vi "Monitor DI Port 1.vi"(8 "Error in":errorcluster, 10 "Sequence Context In":refnum<k7>, 11 "DI_Port1_in":i32) -> (0 "error out":errorcluster)   [LabVIEW 2023]
uses:
  442f22da-24f2-4adb-9ca8-d01af5e2a905.vi
  <userlib>/DAQNavi Polymorphic VI/read/DAQNavi Read (Digital U8 1Chan 1Samp).vi
  <vilib>/addons/TestStand/_TSUtility.llb/TestStand - Set Property Value (Boolean).vi
  <vilib>/addons/TestStand/_TSUtility.llb/TestStand - Get Property Value (Boolean).vi
panel:
  out "Spare":bool
  out "Mouting close-":bool
  out "Cass Code Bit 3":bool
  out "Cass Code Bit 2":bool
  out "Cass Code Bit 1":bool
  out "Cass Code Bit 0":bool
  out "Second safety":bool
  out "First Safety":bool
  out "DI_Port1_Out":i32
  in  "stop":bool
  # "Port 0\nInversed Bits are : 4,5,6,7\nPort 1\nInversed Bits are : 0,1,6\nThis is set in Navigator"
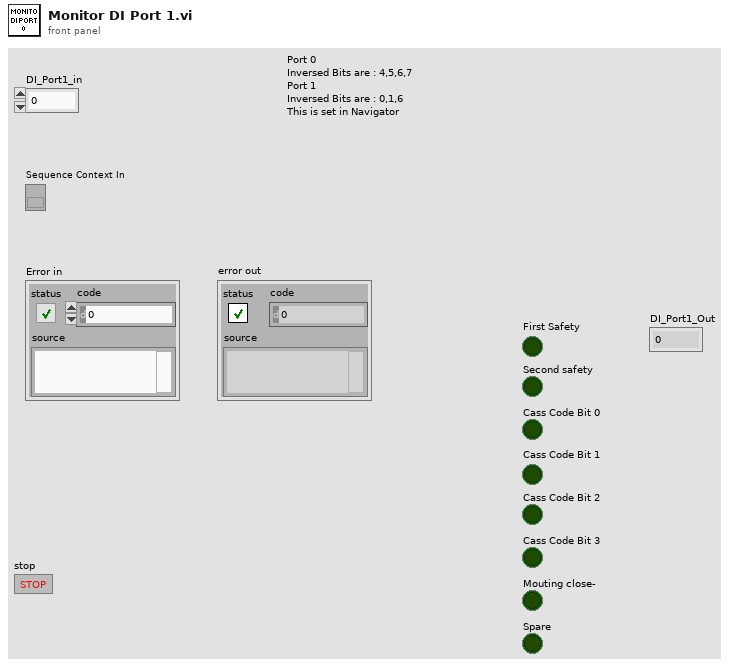
[diagram p1: front panel]
types:
  T1 = typedef "TestStand - Status Monitor.ctl" = cluster{"Sequence Context":refnum<k7>, "Execution":refnum<k7>, "Termination Monitor":refnum<k7>}
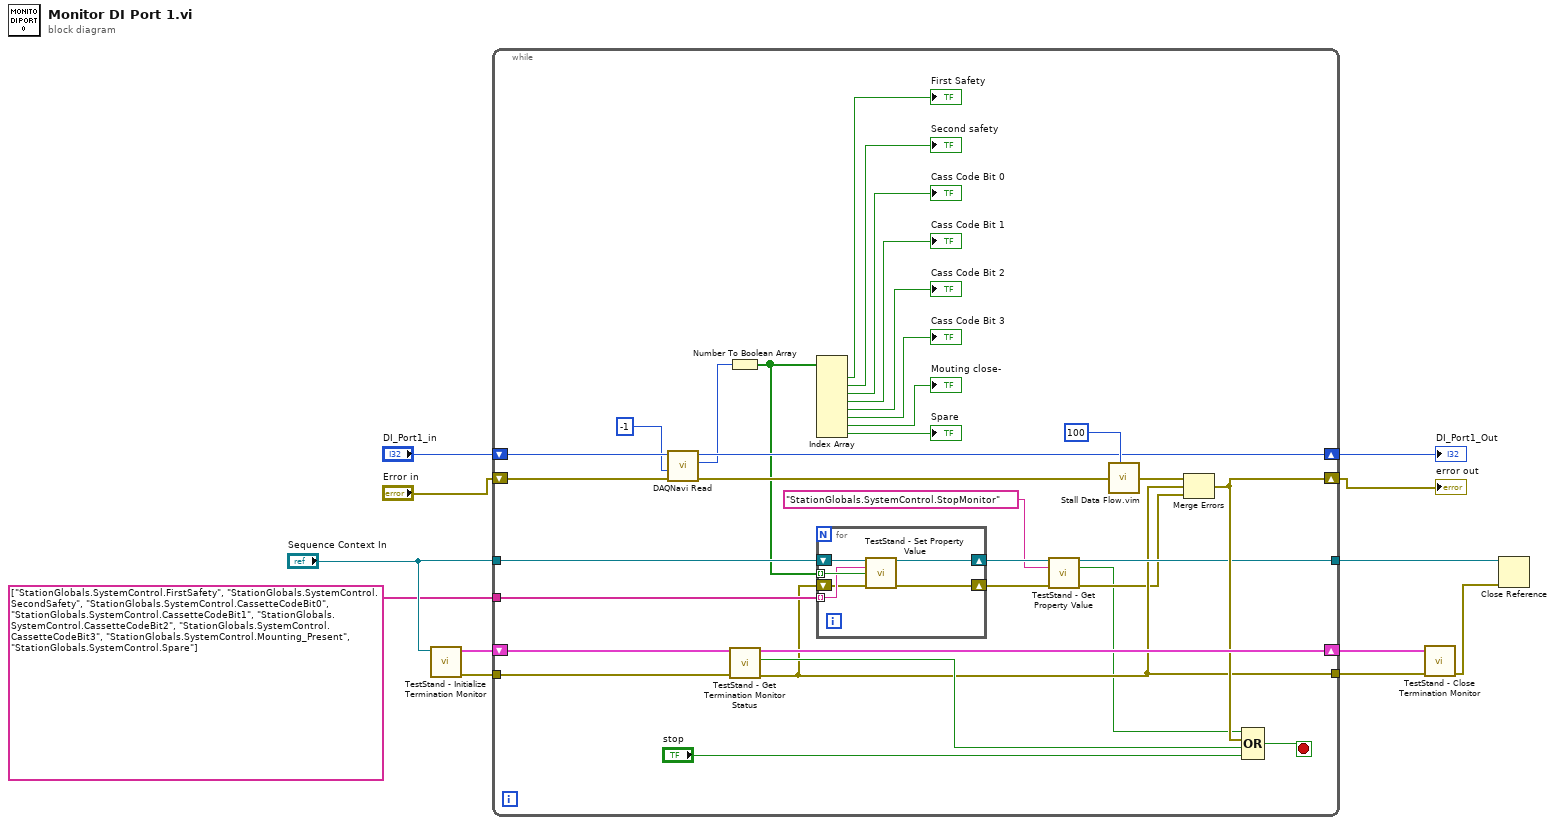
[diagram p0: block diagram]
diagram:
  n1 = call <vilib>:"TestStand - Initialize Termination Monitor.vi"("Sequence Context In"="Sequence Context In") -> ("error out"=w8:errorcluster, "Status Monitor Out"=w9:T1)  [unwired: 9 in]
  n2 = while {
    shift-right: [w41] -> w10
    shift-left: "DI_Port1_in" -> [w44]
    shift-right: [w31] -> w7
    shift-left: "Error in" -> [w43]
    shift-right: [w37] -> w3
    shift-left: w9 -> [w38]
    tunnel: w8 -> [w36]
    tunnel: [w17] -> w4
    tunnel: "Sequence Context In" -> [w30]
    tunnel: [w18] -> w5
    tunnel: string[] ["StationGlobals.SystemControl.FirstSafety", "StationGlobals.SystemControl.SecondSafety", "StationGlobals.SystemControl.CassetteCodeBit0", "StationGlobals.SystemControl.CassetteCodeBit1", "StationGlobals.SystemControl.CassetteCodeBit2", "StationGlobals.SystemControl.CassetteCodeBit3", "StationGlobals.SystemControl.Mounting_Present", "StationGlobals.SystemControl.Spare"] ("Lookup String") -> [w29]
    stop <- w34 stop-if-true
    n3 = call-poly <userlib>:"DAQNavi Read.vi"("error in (no error)"=w43, "portBit"=-1, "task in"=w44) -> ("error out"=w42:errorcluster, "data"=w39:u8, "task out"=w41:i32)  [unwired: 1 in, 5 out]
    n4 = Number To Boolean Array(number=w39) -> (Boolean array=w20:bool[])
    n5 = call <vilib>:"TestStand - Get Termination Monitor Status.vi"("error in (no error)"=w36, "Status Monitor In"=w38) -> ("error out"=w17:errorcluster, "Terminating or Aborting"=w32:bool, "Status Monitor Out"=w37:T1)  [unwired: 7 in]
    n6 = Index Array(array=w20) -> (element #1=→"First Safety":bool, element #2=→"Second safety":bool, element #3=→"Cass Code Bit 0":bool, element #4=→"Cass Code Bit 1":bool, element #5=→"Cass Code Bit 2":bool, element #6=→"Cass Code Bit 3":bool, element #7=→"Mouting close-":bool, element #8=→"Spare":bool)  [unwired: 8 in]
    n7 = for {
      shift-right: [w50] -> w19
      shift-left: w30 -> [w51]
      tunnel: w20 -> [w49] mode=indexing
      tunnel: w29 -> [w48] mode=indexing
      shift-right: [w46] -> w16
      shift-left: w17 -> [w47]
      n8 = call-poly <vilib>:"TestStand - Set Property Value.vi"("Sequence Context In"=w51, "Lookup String"=w48, "New Value"=w49, "error in (no error)"=w47) -> ("Sequence Context Out"=w50:refnum<k7>, "error out"=w46:errorcluster)  [unwired: 10 in]
    }
    n9 = call-poly <vilib>:"TestStand - Get Property Value.vi"("Sequence Context In"=w19, "Lookup String"="StationGlobals.SystemControl.StopMonitor", "error in (no error)"=w16) -> ("Sequence Context Out"=w18:refnum<k7>, "Value"=w13:bool, "error out"=w15:errorcluster)  [unwired: 10 in]
    n10 = call "Stall Data Flow.vim"("value in"=w42, "milliseconds to wait"=u32 100) -> ("value out"=w35:errorcluster)  [unwired: 1 out]
    n11 = Merge Errors(w35, w17, w15) -> (w31:errorcluster)
    n12 = Compound Arithmetic op=OR(w13, w31, w32, "stop") -> (w34:bool)
  }
  "error out" <- w7
  "DI_Port1_Out" <- w10
  n13 = call <vilib>:"TestStand - Close Termination Monitor.vi"("error in (no error)"=w4, "Status Monitor In"=w3) -> ("error out"=w2:errorcluster)  [unwired: 9 in]
  n14 = Close Reference(reference=w5, error in (no error)=w2) -> ()  [unwired: 1 out]
